vi "PXI-Init AO Buffer.vi"(8 "error in (no error)":errorcluster) -> (0 "error out":errorcluster)   [LabVIEW 2015]
uses:
  PXI Globals.vi
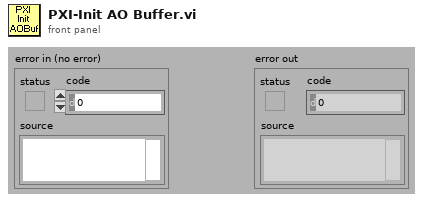
[diagram p1: front panel]
types:
  T1 = typedef "Task Struct.ctl" = cluster{"Task name":string, "Task":refnum<k21>, "Dual-channel task?":bool, "Regenerate?":bool, "Clear?":bool}
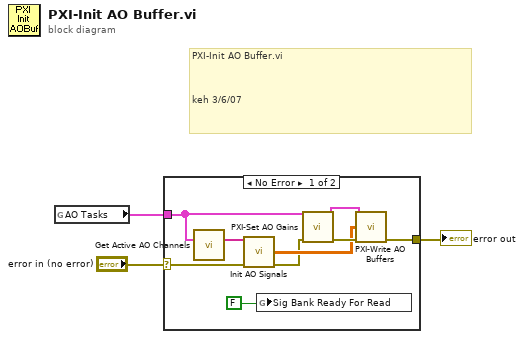
[diagram p0: block diagram]
diagram:
  # "PXI-Init AO Buffer.vi\n\n\n\nkeh 3/6/07"
  n1 = global read "PXI Globals.vi" "AO Tasks"() -> (w3:T1[])
  n2 = case shown="No Error" "error in (no error)" {
    selector: "error in (no error)" -> [w11 w13]
    tunnel: w3 -> [w6 _]
    tunnel: [w10 w13] -> w1
    frame No Error {
      n3 = call "Get Active AO Channels.vi"("AO Tasks"=w6) -> ("AO Channel Names"=w12:string[])  [unwired: 13 in, 1 out]
      n4 = call "Init AO Signals.vi"("AO Tasks"=w12, "error in (no error)"=w11) -> ("AO Waveforms"=w5:dbl[][], "error out"=w4:errorcluster)  [unwired: 12 in]
      n5 = global write "PXI Globals.vi" "Sig Bank Ready For Read"(FALSE) -> ()
      n6 = call "PXI-Set AO Gains.vi"("error in (no error)"=w4, "AO Tasks"=w6) -> ("error out"=w7:errorcluster, "AO Tasks out"=w8:T1[])  [unwired: 8 in]
      n7 = call "PXI-Write AO Buffers.vi"("AO Tasks"=w8, "AO Waveforms"=w5, "error in (no error)"=w7) -> ("error out"=w10:errorcluster)  [unwired: 11 in, 1 out]
    }
    frame Error {
    }
  }
  "error out" <- w1
